vi "WriteSignalToTXT.vi"(8 "error in":errorcluster, 10 "signal in":waveform(dbl), 11 "file path in":path) -> (0 "error out":errorcluster, 3 "file path out":path)   [LabVIEW 2025]
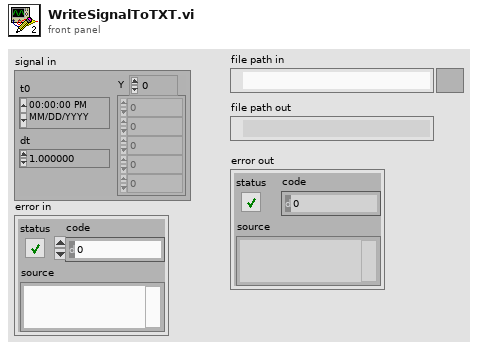
[diagram p1: front panel]
types:
  T1 = enum16{"open", "replace", "create", "open or create", "replace or create", "replace or create with confirmation"}
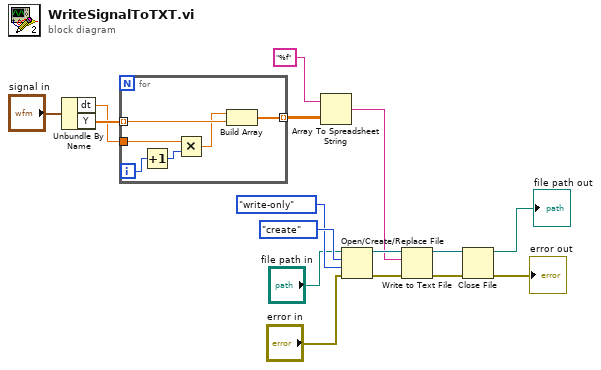
[diagram p0: block diagram]
diagram:
  n1 = Unbundle By Name("signal in") -> ("dt"=w9:dbl, "Y"=w10:dbl[])
  n2 = for {
    tunnel: w10 -> [w21] mode=indexing
    tunnel: w9 -> [w19]
    tunnel: [w17] -> w8 mode=indexing
    i -> [w22]
    n3 = Increment(x=w22) -> (x+1=w20:i32)
    n4 = Multiply(x=w19, y=w20) -> (x*y=w18:dbl)
    n5 = Build Array(w18, w21) -> (w17:dbl[])
  }
  n6 = Array To Spreadsheet String(array=w8, 3:"%f" ("format string")) -> (spreadsheet string=w7:string)  [unwired: 1 in]
  n7 = Open/Create/Replace File(file path (use dialog)="file path in", error in="error in", operation (0:open)=T1."create", access (0:read/write)=enum16{"read/write", "read-only", "write-only"}."write-only") -> (refnum out=w14:refnum<file>, error out=w13:errorcluster)  [unwired: 2 in, 1 out]
  n8 = Write to Text File(file (use dialog)=w14, text=w7, error in=w13) -> (refnum out=w6:refnum<file>, error out=w5:errorcluster)  [unwired: 1 in, 1 out]
  n9 = Close File(refnum=w6, error in=w5) -> (path=→"file path out":path, error out=→"error out":errorcluster)
